vi "robo BRAÇO.vi"   [LabVIEW 2016]
uses:
  <vilib>/NXT/Subs/LVHSConnector.ctl
  <vilib>/NXT/LegoClasses/BrickReference/BrickReference.lvclass
  <vilib>/NXT/Block Support/NXT_OutputPort.ctl
  <vilib>/NXT/Block Support/NXT_InputPort.ctl
  <vilib>/NXT/Block Support/NXT_ButtonSelector.ctl
  <vilib>/NXT/Dual Mode Library/Waits/Wait_Num.vi
  <vilib>/NXT/Dual Mode Library/Sensors/EV3_Color_Reflect.vi
  <vilib>/NXT/Dual Mode Library/Sound/Tone.vi
  <vilib>/NXT/NXTIO Xnodes/NXTIONodeSubVIs/NXTMoveMotors.vi
  <vilib>/NXT/Dual Mode Library/Sensors/EV3_Ultrasonic_CM.vi
  <vilib>/NXT/NXTIO Xnodes/NXTIONodeSubVIs/NXTStopMotors.vi
  <vilib>/NXT/Dual Mode Library/Sensors/readNXTButton.vi
  <vilib>/NXT/NXTIO Xnodes/AddressXNode/NXTIOAddress.xnode
  <vilib>/NXT/NXTIO Xnodes/NXTIOXNode/NXTIO.xnode
types:
  T1 = typedef "LVHSConnector.ctl" = refnum<class "BrickReference.lvclass">
  T2 = typedef "NXT_OutputPort.ctl" = u8
  T3 = typedef "NXT_ButtonSelector.ctl" = u16
  T4 = typedef "NXT_InputPort.ctl" = u32
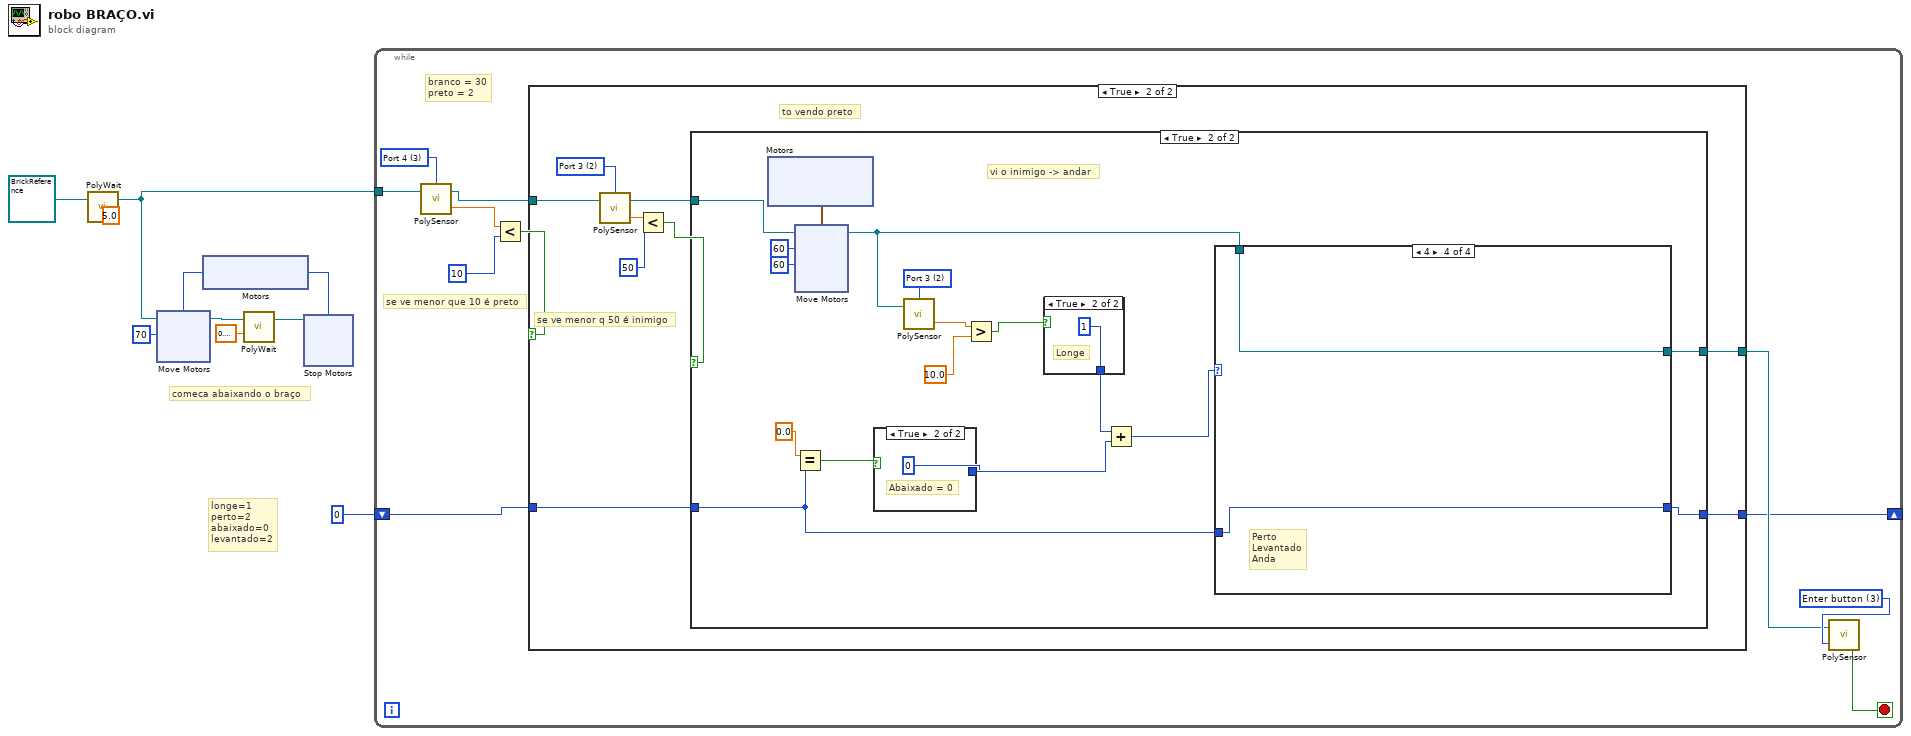
[diagram p0: block diagram]
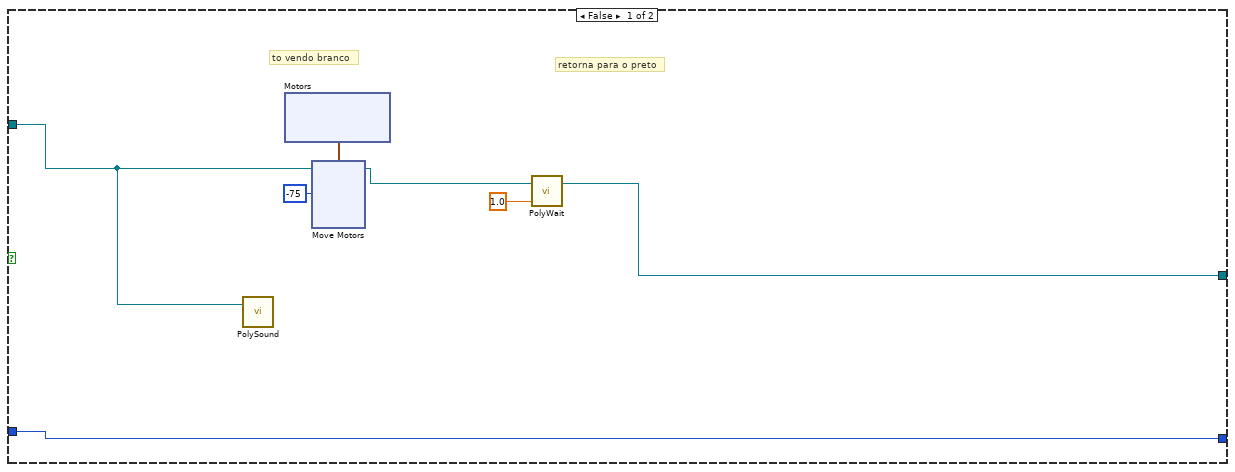
[diagram p2: hidden frame]
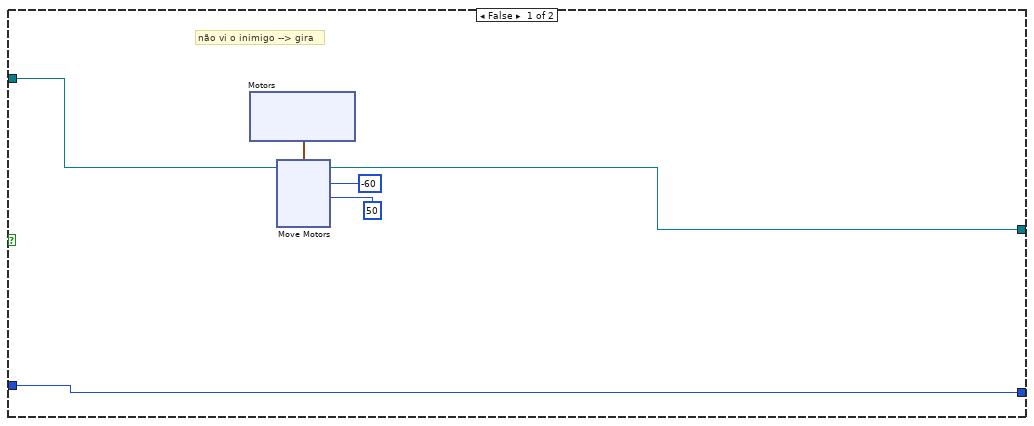
[diagram p3: hidden frame]
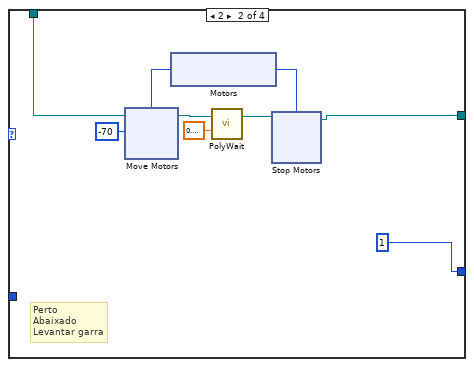
[diagram p5: hidden frame]
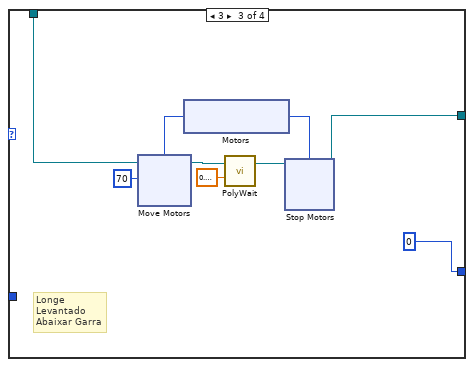
[diagram p6: hidden frame]
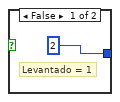
[diagram p7: hidden frame]
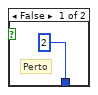
[diagram p8: hidden frame]
diagram:
  # "comeca abaixando o braço"
  # "longe=1\nperto=2\nabaixado=0\nlevantado=2"
  n1 = call-poly <vilib>:"PolyWait.vi"("Time (1 sec)"=sgl 5.0, "NXT/EV3"=T1 refnum ("y")) -> ("NXT/EV3"=w4:T1)  [unwired: 2 in]
  n2 = xnode "Motors"() -> ("Motor"=w2:T2)
  n3 = xnode "Move Motors"("Power/Speed 1"=i8 70, "Motors"=w2, "NXT/EV3"=w4) -> ("NXT/EV3"=w5:T1)
  n4 = call-poly <vilib>:"PolyWait.vi"("Time (1 sec)"=sgl 0.2, "NXT/EV3"=w5) -> ("NXT/EV3"=w6:T1)  [unwired: 2 in]
  n5 = xnode "Stop Motors"("Motors"=w2, "NXT/EV3"=w6) -> ()  [unwired: 1 out]
  n6 = while {
    tunnel: w4 -> [w19]
    shift-right: [w12] -> _
    shift-left: 0 -> [w16]
    stop <- w14 stop-if-true
    w15 = T3 3 items=["Enter button"=3, "Left button"=2, "Right button"=1, "Up Button"=4, "Down Button"=5] ("Button (Enter button)")
    w17 = T4 3 items=["Port 1", "Port 2", "Port 3", "Port 4"] ("Port (Port 1)")
    # "se ve menor que 10 é preto"
    # "branco = 30\npreto = 2"
    n7 = call-poly <vilib>:"PolySensor.vi"("NXT/EV3"=w19, "Port (Port 1)"=w17) -> ("Scaled Value"=w20:sgl, "NXT/EV3"=w18:T1)  [unwired: 1 in]
    n8 = Less?(x=w20, y=10) -> (x < y?=w11:bool)
    n9 = case shown="True" w11 {
      tunnel: w18 -> [w21 w45]
      tunnel: w16 -> [w22 w42]
      tunnel: [w23 w41] -> w13
      tunnel: [w22 w40] -> w12
      frame False {
        w26 = i8 -75 ("Power/Speed 2")
        # "retorna para o preto"
        # "to vendo branco"
        n10 = call-poly <vilib>:"PolySound.vi"("NXT/EV3"=w21) -> ()  [unwired: 3 in, 1 out]
        n11 = xnode "Motors"() -> ("Motor"=w27:cluster{"Port":T2, "Port":T2})
        n12 = xnode "Move Motors"("Power/Speed 2"=w26, "Power/Speed 1"=w26, "Motors"=w27, "NXT/EV3"=w21) -> ("NXT/EV3"=w24:T1)
        n13 = call-poly <vilib>:"PolyWait.vi"("Time (1 sec)"=sgl 1.0, "NXT/EV3"=w24) -> ("NXT/EV3"=w23:T1)  [unwired: 2 in]
      }
      frame True {
        w44 = T4 2 items=["Port 1", "Port 2", "Port 3", "Port 4"] ("Port (Port 1)")
        # "to vendo preto"
        # "se ve menor q 50 é inimigo"
        n14 = call-poly <vilib>:"PolySensor.vi"("NXT/EV3"=w45, "Port (Port 1)"=w44) -> ("Centimeters"=w38:sgl, "NXT/EV3"=w43:T1)  [unwired: 1 in]
        n15 = Less?(x=w38, y=50) -> (x < y?=w37:bool)
        n16 = case shown="True" w37 {
          tunnel: w43 -> [w49 w61]
          tunnel: w42 -> [w47 w65]
          tunnel: [w48 w66] -> w41
          tunnel: [w47 w64] -> w40
          frame False {
            # "não vi o inimigo --> gira"
            n17 = xnode "Motors"() -> ("Motor"=w50:cluster{"Port":T2, "Port":T2})
            n18 = xnode "Move Motors"("Power/Speed 2"=i8 50, "Power/Speed 1"=i8 -60 ("Power/Speed 2"), "Motors"=w50, "NXT/EV3"=w49) -> ("NXT/EV3"=w48:T1)
          }
          frame True {
            w74 = T4 2 items=["Port 1", "Port 2", "Port 3", "Port 4"] ("Port (Port 1)")
            # "vi o inimigo -> andar"
            n19 = xnode "Motors"() -> ("Motor"=w77:cluster{"Port":T2, "Port":T2})
            n20 = xnode "Move Motors"("Power/Speed 2"=i8 60, "Power/Speed 1"=i8 60, "Motors"=w77, "NXT/EV3"=w61) -> ("NXT/EV3"=w72:T1)
            n21 = Equal?(x=0.0, y=w65) -> (x = y?=w68:bool)
            n22 = case shown="True" w68 {
              tunnel: [2 0] -> w69
              frame False {
                # "Levantado = 1"
              }
              frame True {
                # "Abaixado = 0"
              }
            }
            n23 = call-poly <vilib>:"PolySensor.vi"("NXT/EV3"=w72, "Port (Port 1)"=w74) -> ("Centimeters"=w75:sgl)  [unwired: 1 in, 1 out]
            n24 = Greater?(x=w75, y=sgl 10.0) -> (0:w73:bool)
            n25 = case shown="True" w73 {
              tunnel: [2 1] -> w70
              frame False {
                # "Perto"
              }
              frame True {
                # "Longe"
              }
            }
            n26 = Add(x=w70, y=w69) -> (x+y=w67:i32)
            n27 = case shown="4" w67 {
              tunnel: w72 -> [w79 w80 w102 w123]
              tunnel: [w79 w81 w101 w123] -> w66
              tunnel: [w78 1 0 w122] -> w64
              tunnel: w65 -> [w78 _ _ w122]
              frame 1, Default {
                # "Longe\nAbaixado\nAnda"
              }
              frame 2 {
                # "Perto\nAbaixado\nLevantar garra"
                n28 = xnode "Motors"() -> ("Motor"=w86:T2)
                n29 = xnode "Move Motors"("Power/Speed 1"=i8 -70, "Motors"=w86, "NXT/EV3"=w80) -> ("NXT/EV3"=w84:T1)
                n30 = call-poly <vilib>:"PolyWait.vi"("Time (1 sec)"=sgl 0.3, "NXT/EV3"=w84) -> ("NXT/EV3"=w83:T1)  [unwired: 2 in]
                n31 = xnode "Stop Motors"("Motors"=w86, "NXT/EV3"=w83) -> ("NXT/EV3"=w81:T1)
              }
              frame 3 {
                # "Longe\nLevantado\nAbaixar Garra"
                n32 = xnode "Motors"() -> ("Motor"=w103:T2)
                n33 = xnode "Move Motors"("Power/Speed 1"=i8 70, "Motors"=w103, "NXT/EV3"=w102) -> ("NXT/EV3"=w105:T1)
                n34 = call-poly <vilib>:"PolyWait.vi"("Time (1 sec)"=sgl 0.3, "NXT/EV3"=w105) -> ("NXT/EV3"=w106:T1)  [unwired: 2 in]
                n35 = xnode "Stop Motors"("Motors"=w103, "NXT/EV3"=w106) -> ("NXT/EV3"=w101:T1)
              }
              frame 4 {
                # "Perto\nLevantado\nAnda"
              }
            }
          }
        }
      }
    }
    n36 = call-poly <vilib>:"PolySensor.vi"("Button (Enter button)"=w15, "NXT/EV3"=w13) -> ("Yes/No"=w14:bool)  [unwired: 1 in, 1 out]
  }
